vi "Funnel Path Points.vi"(8 "Smooth Segments":dbl, 11 "Commands":T1(array[cluster])) -> (0 "Array 2":cluster{"X":dbl, "Y":dbl}[](array[cluster]), 2 "Commands":string[](array[string]), 3 "Array":cluster{"X":dbl, "Y":dbl}[][](array[cluster]))   [LabVIEW 2019]
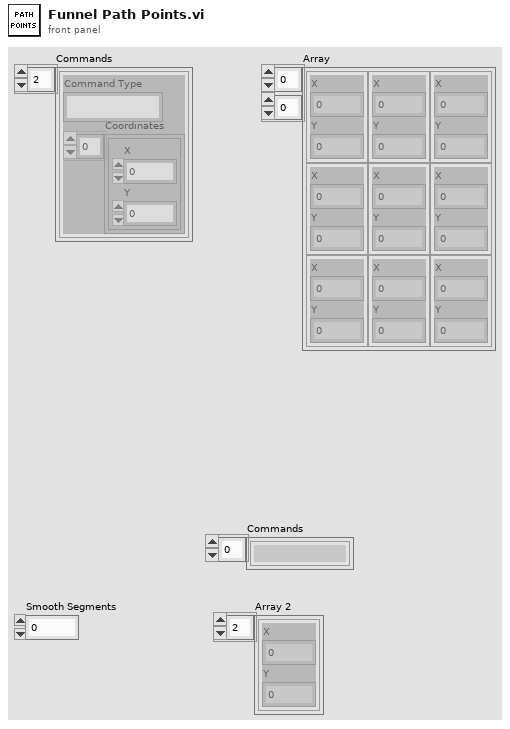
[diagram p1: front panel]
types:
  T1 = cluster{"Command Type":string, "Coordinates":cluster{"X":dbl, "Y":dbl}[]}[]
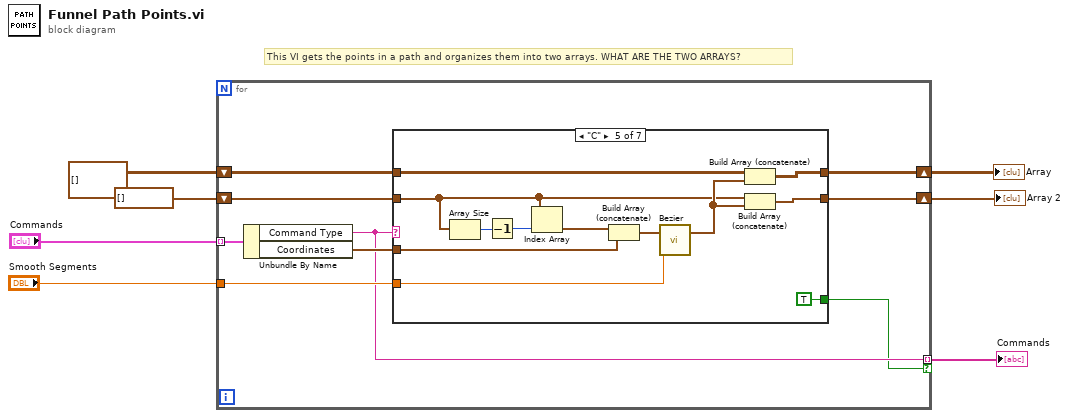
[diagram p0: block diagram]
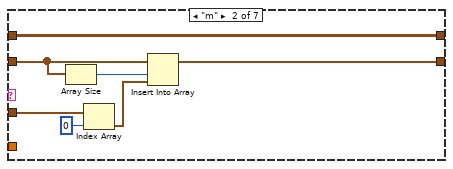
[diagram p3: hidden frame]
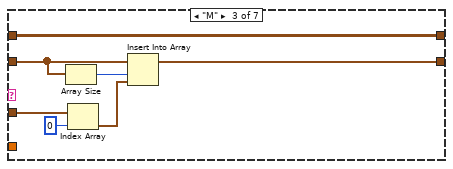
[diagram p4: hidden frame]
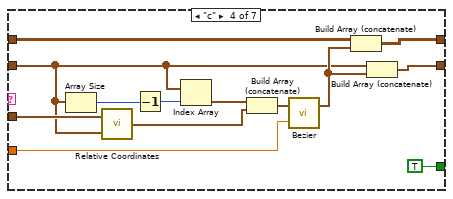
[diagram p5: hidden frame]
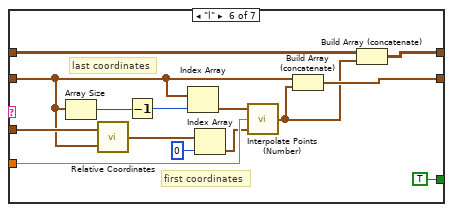
[diagram p6: hidden frame]
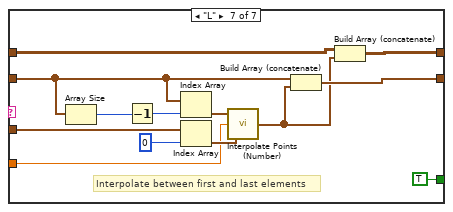
[diagram p7: hidden frame]
diagram:
  # "This VI gets the points in a path and organizes them into two arrays. WHAT ARE THE TWO ARRAYS?"
  n1 = for {
    tunnel: "Commands" -> [w16] mode=indexing
    shift-right: [w10] -> w3
    shift-left: cluster{"X":dbl, "Y":dbl}[] [] -> [w13]
    tunnel: "Smooth Segments" -> [w11]
    shift-right: [w15] -> w1
    shift-left: cluster{"X":dbl, "Y":dbl}[][] [] -> [w12]
    tunnel: [w9] -> w2 mode=indexing if=w8
    n2 = Unbundle By Name(w16) -> ("Command Type"=w9:string, "Coordinates"=w14:cluster{"X":dbl, "Y":dbl}[])
    n3 = case shown="\"C\"" w9 {
      tunnel: w14 -> [_ w20 w30 w41 w47 w68 w84]
      tunnel: w13 -> [w18 w22 w27 w35 w48 w66 w80]
      tunnel: [w18 w23 w28 w36 w51 w71 w79] -> w10
      tunnel: w11 -> [_ _ _ w34 w53 w61 w76]
      tunnel: [w17 w19 w29 w37 w52 w65 w74] -> w15
      tunnel: w12 -> [w17 w19 w29 w40 w56 w67 w73]
      tunnel: [_ _ _ TRUE TRUE TRUE TRUE] -> w8
      frame "other letters", Default {
      }
      frame "m" {
        n4 = Array Size(array=w22) -> (size(s)=w25:i32)
        n5 = Index Array(array=w20, index=0) -> (element=w24:cluster{"X":dbl, "Y":dbl})
        n6 = Insert Into Array(array=w22, index=w25, new element=w24) -> (w23:cluster{"X":dbl, "Y":dbl}[])
      }
      frame "M" {
        n7 = Array Size(array=w27) -> (size(s)=w31:i32)
        n8 = Index Array(array=w30, index=0) -> (element=w26:cluster{"X":dbl, "Y":dbl})
        n9 = Insert Into Array(array=w27, index=w31, new element=w26) -> (w28:cluster{"X":dbl, "Y":dbl}[])
      }
      frame "c" {
        n10 = Array Size(array=w35) -> (size(s)=w43:i32)
        n11 = call "Relative Coordinates.vi"("All Coordinates"=w35, "Command Coordinates"=w41) -> ("Adjusted Command Coordinates"=w44:cluster{"X":dbl, "Y":dbl}[])
        n12 = Decrement(x=w43) -> (x-1=w42:i32)
        n13 = Index Array(array=w35, index=w42) -> (element=w45:cluster{"X":dbl, "Y":dbl})
        n14 = Build Array (concatenate)(w45, w44) -> (w39:cluster{"X":dbl, "Y":dbl}[])
        n15 = call "Bezier.vi"("Segments"=w34, "Parameters"=w39) -> ("Coordinate Array"=w38:cluster{"X":dbl, "Y":dbl}[])  [unwired: 1 out]
        n16 = Build Array (concatenate)(w40, w38) -> (w37:cluster{"X":dbl, "Y":dbl}[][])
        n17 = Build Array (concatenate)(w35, w38) -> (w36:cluster{"X":dbl, "Y":dbl}[])
      }
      frame "C" {
        n18 = Array Size(array=w48) -> (size(s)=w57:i32)
        n19 = Decrement(x=w57) -> (x-1=w49:i32)
        n20 = Index Array(array=w48, index=w49) -> (element=w50:cluster{"X":dbl, "Y":dbl})
        n21 = Build Array (concatenate)(w50, w47) -> (w55:cluster{"X":dbl, "Y":dbl}[])
        n22 = call "Bezier.vi"("Segments"=w53, "Parameters"=w55) -> ("Coordinate Array"=w54:cluster{"X":dbl, "Y":dbl}[])  [unwired: 1 out]
        n23 = Build Array (concatenate)(w56, w54) -> (w52:cluster{"X":dbl, "Y":dbl}[][])
        n24 = Build Array (concatenate)(w48, w54) -> (w51:cluster{"X":dbl, "Y":dbl}[])
      }
      frame "l" {
        # "first coordinates"
        # "last coordinates"
        n25 = Array Size(array=w66) -> (size(s)=w69:i32)
        n26 = call "Relative Coordinates.vi"("All Coordinates"=w66, "Command Coordinates"=w68) -> ("Adjusted Command Coordinates"=w70:cluster{"X":dbl, "Y":dbl}[])
        n27 = Decrement(x=w69) -> (x-1=w64:i32)
        n28 = Index Array(array=w66, index=w64) -> (element=w62:cluster{"X":dbl, "Y":dbl})
        n29 = Index Array(array=w70, index=0) -> (element=w59:cluster{"X":dbl, "Y":dbl})
        n30 = call "Interpolate Points (Number).vi"("End Point"=w59, "Number of Points"=w61, "Start Point"=w62) -> ("Output Point Array"=w60:cluster{"X":dbl, "Y":dbl}[])
        n31 = Build Array (concatenate)(w66, w60) -> (w71:cluster{"X":dbl, "Y":dbl}[])
        n32 = Build Array (concatenate)(w67, w60) -> (w65:cluster{"X":dbl, "Y":dbl}[][])
      }
      frame "L" {
        # "Interpolate between first and last elements"
        n33 = Array Size(array=w80) -> (size(s)=w82:i32)
        n34 = Decrement(x=w82) -> (x-1=w81:i32)
        n35 = Index Array(array=w80, index=w81) -> (element=w78:cluster{"X":dbl, "Y":dbl})
        n36 = Index Array(array=w84, index=0) -> (element=w77:cluster{"X":dbl, "Y":dbl})
        n37 = call "Interpolate Points (Number).vi"("End Point"=w77, "Number of Points"=w76, "Start Point"=w78) -> ("Output Point Array"=w72:cluster{"X":dbl, "Y":dbl}[])
        n38 = Build Array (concatenate)(w80, w72) -> (w79:cluster{"X":dbl, "Y":dbl}[])
        n39 = Build Array (concatenate)(w73, w72) -> (w74:cluster{"X":dbl, "Y":dbl}[][])
      }
    }
  }
  "Array" <- w1
  "Array 2" <- w3
  "Commands" <- w2
